vi "chooseParametersFromFiles.vi"(0 "Game in":refnum<class "Game.lvclass">, 1 "MainGameConfigs":T1={"SSL UDP RX"={"Local IP:"="", "Port"=10002, "Server IP:"="224.0.0.1"}, "RefBox UDP RX"={"Local IP:"="", "Port"=10003, "Server IP:"="224.5.23.2"}, "Com UDP"={"UDP GrSim TX"=TRUE, "Address:"="172.31.17.157", "Port:"=20011}, "Command"="Auto", "Goalie"="0", "Side"=enum."Esquerdo", "Team"=enum."Azul"}, 5 "error in (no error)":errorcluster, 7 "ParametersFromFile":T4) -> (14 "Game out":refnum<class "Game.lvclass">, 15 "MainGameConfigs out":T1={"SSL UDP RX"={"Local IP:"="", "Port"=10002, "Server IP:"="224.0.0.1"}, "RefBox UDP RX"={"Local IP:"="", "Port"=10003, "Server IP:"="224.5.23.2"}, "Com UDP"={"UDP GrSim TX"=TRUE, "Address:"="172.31.17.157", "Port:"=20011}, "Command"="Auto", "Goalie"="0", "Side"=enum."Esquerdo", "Team"=enum."Azul"}, 19 "error out":errorcluster)   [LabVIEW 2020, in "Game.lvclass"]
uses:
  Game.lvclass
  ParametersFromFile.ctl
  MainGameConfig.ctl
  Controls/vision_control.ctl
  Controls/ComUDP.ctl
  Utilities_class/Utilities.lvclass
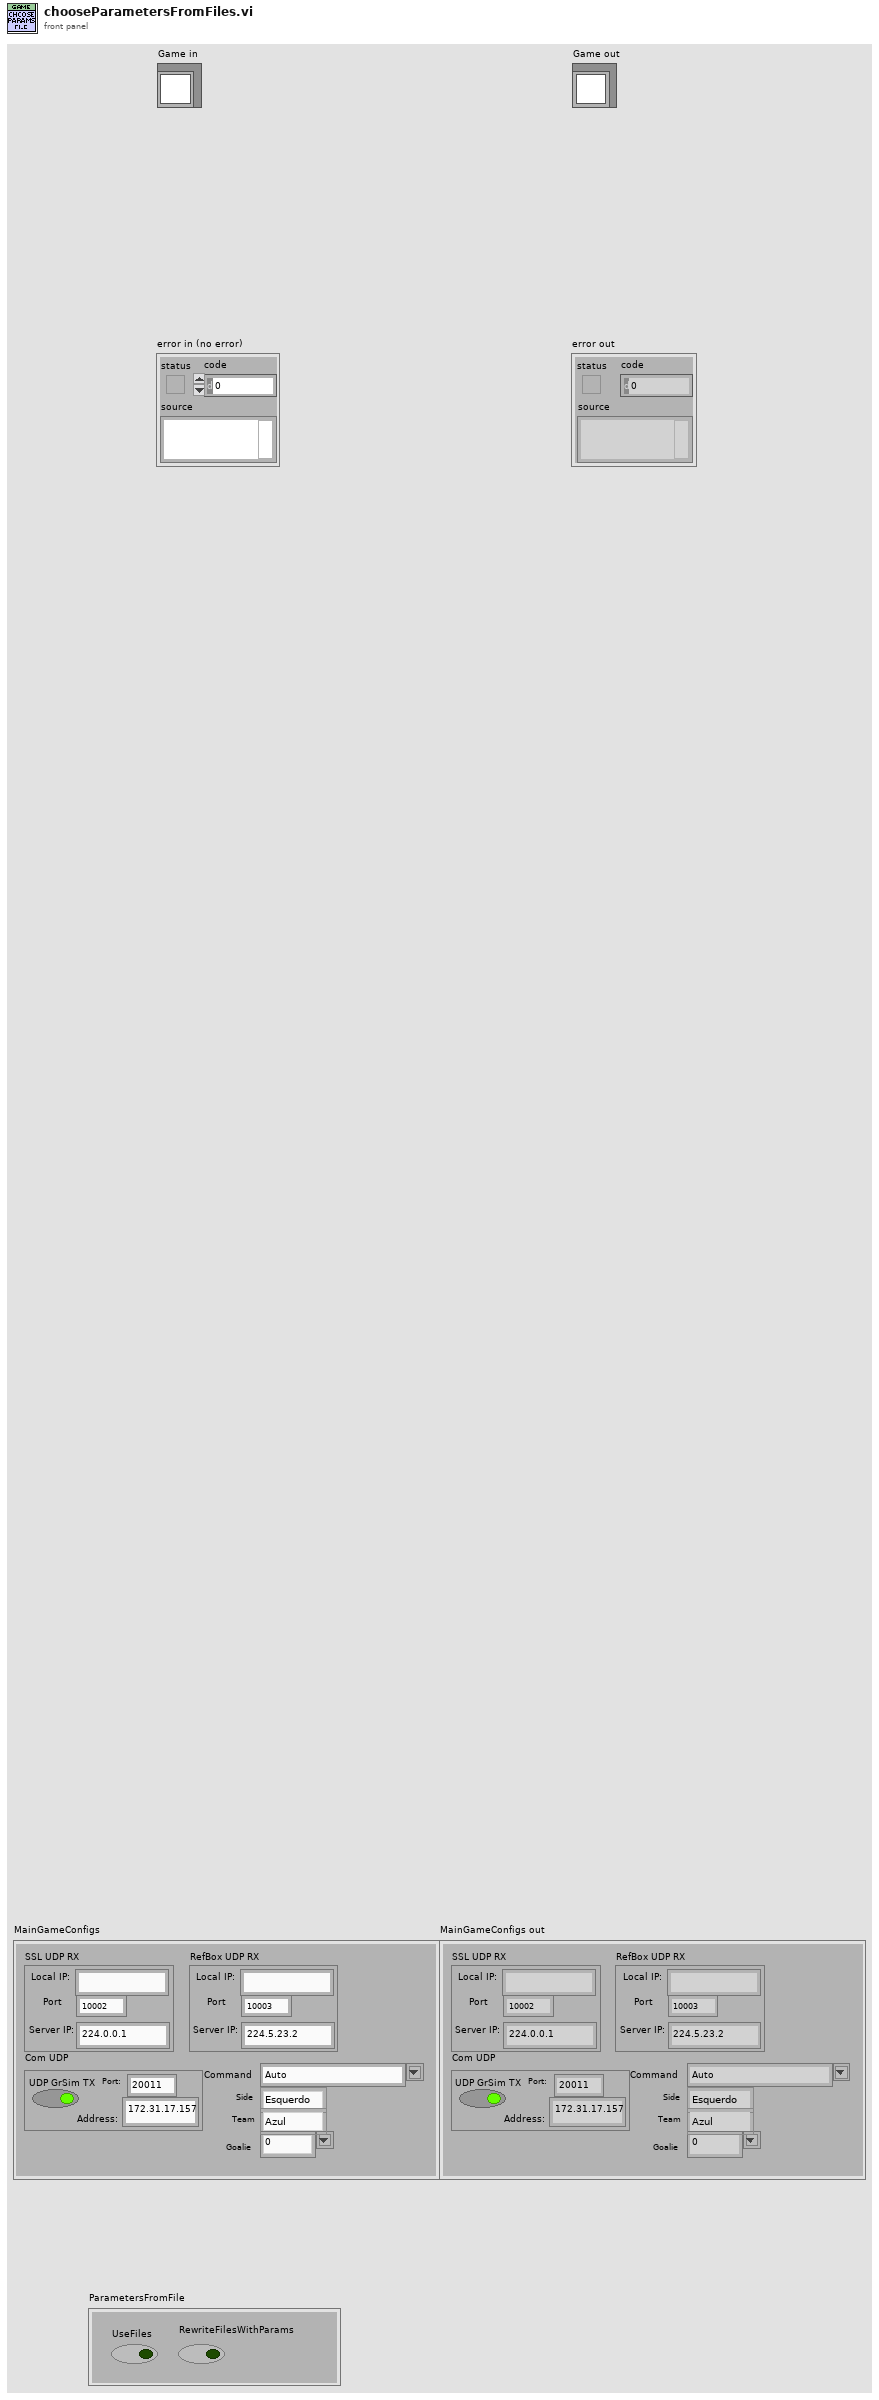
[diagram p1: front panel]
types:
  T1 = typedef "MainGameConfig.ctl" = cluster{"SSL UDP RX":T2, "RefBox UDP RX":T2, "Com UDP":T3, "Command":string, "Goalie":string, "Side":enum16{"Esquerdo", "Direito"}, "Team":enum16{"Azul", "Amarelo"}}
  T2 = typedef "vision_control.ctl" = cluster{"Local IP:":string, "Port":i32, "Server IP:":string}
  T3 = typedef "ComUDP.ctl" = cluster{"UDP GrSim TX":bool, "Address:":string, "Port:":u16}
  T4 = typedef "ParametersFromFile.ctl" = cluster{"UseFiles":bool, "RewriteFilesWithParams":bool}
  T5 = enum16{"open", "replace", "create", "open or create", "replace or create", "replace or create with confirmation"}
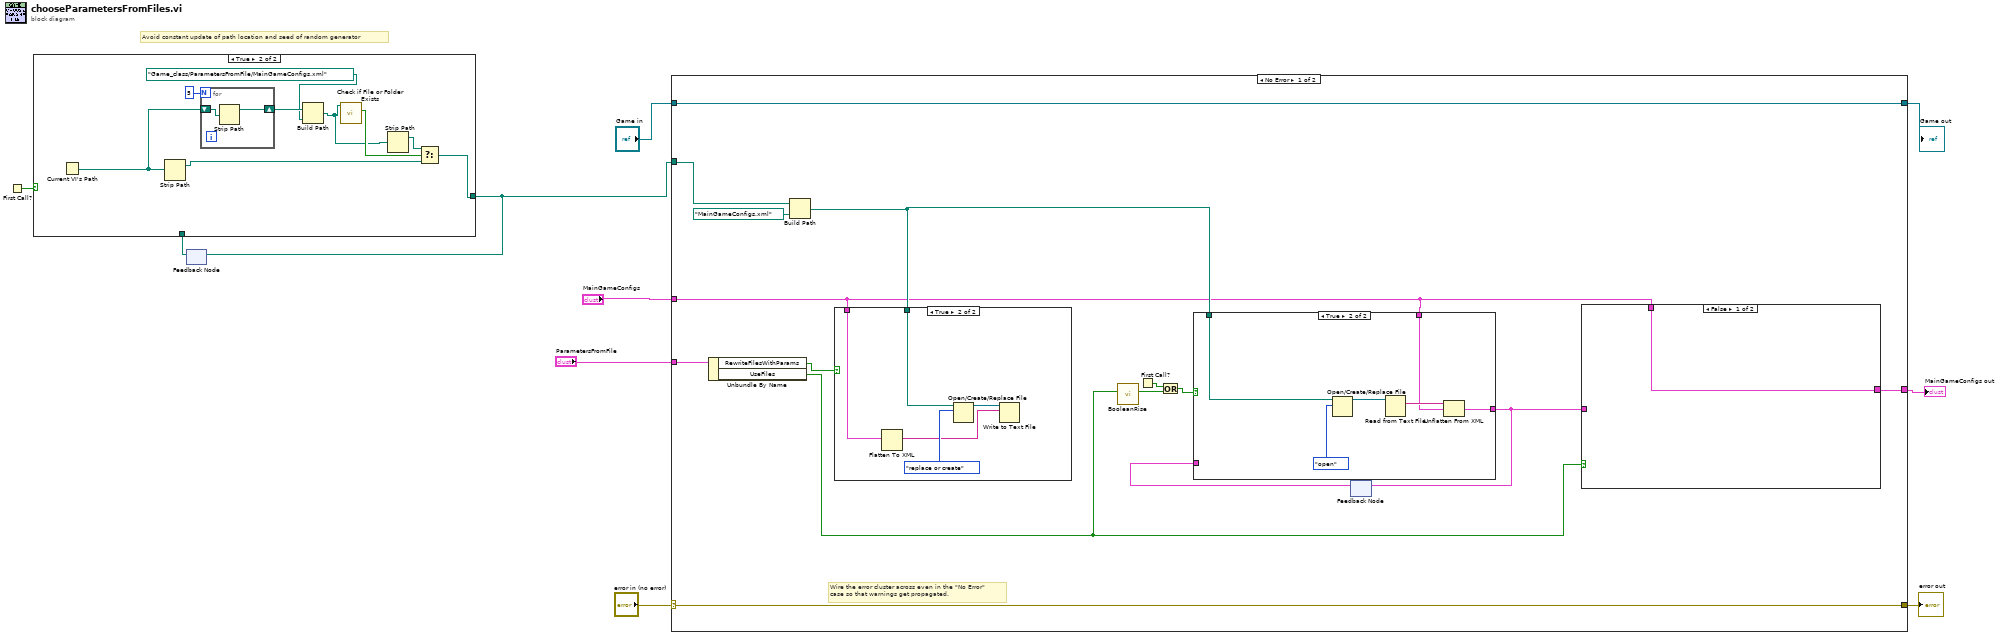
[diagram p0: block diagram]
diagram:
  # "Avoid constant update of path location and seed of random generator"
  n1 = First Call?() -> (First Call?: T/F=w3:bool)
  n2 = feedback #1() -> (w5:path)  [unwired: 1 in]
  n3 = case shown="True" w3 {
    tunnel: [w11 w17] -> w4
    tunnel: w5 -> [w11 _]
    frame False {
    }
    frame True {
      n4 = Current VI's Path() -> (path=w12:path)
      n5 = Strip Path(path=w12) -> (stripped path=w15:path)  [unwired: 1 out]
      n6 = for {
        N: 5 -> [_]
        shift-right: [w21] -> w19
        shift-left: w12 -> [w22]
        n7 = Strip Path(path=w22) -> (stripped path=w21:path)  [unwired: 1 out]
      }
      n8 = Build Path(base path=w19, name or relative path=path "Game_class/ParametersFromFile/MainGameConfigs.xml") -> (appended path=w14:path)
      n9 = call <vilib>:"Check if File or Folder Exists.vi"("path"=w14) -> ("file or folder exists?"=w16:bool)  [unwired: 8 in, 2 out]
      n10 = Strip Path(path=w14) -> (stripped path=w13:path)  [unwired: 1 out]
      n11 = Select(t=w13, s=w16, f=w15) -> (s? t:f=w17:path)
    }
  }
  n12 = feedback-in #1(w4) -> ()
  n13 = case shown="No Error" "error in (no error)" {
    selector: "error in (no error)" -> [w36 w53]
    tunnel: [w36 w53] -> w9
    tunnel: [w37 w52] -> w7
    tunnel: "Game in" -> [w37 w52]
    tunnel: "MainGameConfigs" -> [w29 _]
    tunnel: "ParametersFromFile" -> [w33 _]
    tunnel: w4 -> [w34 _]
    tunnel: [w26 _] -> w1
    frame No Error {
      # "Wire the error cluster across even in the \"No Error\"\ncase so that warnings get propagated."
      n14 = Unbundle By Name(w33) -> ("RewriteFilesWithParams"=w32:bool, "UseFiles"=w31:bool)
      n15 = Build Path(base path=w34, name or relative path=path "MainGameConfigs.xml") -> (appended path=w30:path)
      n16 = case shown="True" w32 {
        tunnel: w29 -> [_ w48]
        tunnel: w30 -> [_ w51]
        frame False {
        }
        frame True {
          n17 = Flatten To XML(6:w48) -> (2:w47:string)
          n18 = Open/Create/Replace File(file path (use dialog)=w51, operation (0:open)=T5."replace or create") -> (refnum out=w49:refnum<file>)  [unwired: 4 in, 2 out]
          n19 = Write to Text File(file (use dialog)=w49, text=w47) -> ()  [unwired: 2 in, 3 out]
        }
      }
      n20 = call "BooleanRise.vi"("Boolean in"=w31) -> ("Boolean"=w24:bool)  [unwired: 8 in, 2 out]
      n21 = First Call?() -> (First Call?: T/F=w25:bool)
      n22 = Or(x=w25, y=w24) -> (x .or. y?=w23:bool)
      n23 = feedback #2() -> (w28:T1)  [unwired: 1 in]
      n24 = case shown="True" w23 {
        tunnel: w30 -> [_ w42]
        tunnel: w29 -> [_ w40]
        tunnel: [w38 w39] -> w27
        tunnel: w28 -> [w38 _]
        frame False {
        }
        frame True {
          n25 = Open/Create/Replace File(file path (use dialog)=w42, operation (0:open)=T5."open") -> (refnum out=w44:refnum<file>)  [unwired: 4 in, 2 out]
          n26 = Read from Text File(file (use dialog)=w44) -> (text=w41:string)  [unwired: 3 in, 3 out]
          n27 = Unflatten From XML(xml string=w41, type=w40) -> (value=w39:T1)  [unwired: 1 in, 1 out]
        }
      }
      n28 = feedback-in #2(w27) -> ()
      n29 = case shown="False" w31 {
        tunnel: w29 -> [w45 _]
        tunnel: [w45 w46] -> w26
        tunnel: w27 -> [_ w46]
        frame False {
        }
        frame True {
        }
      }
    }
    frame Error {
    }
  }
  "error out" <- w9
  "Game out" <- w7
  "MainGameConfigs out" <- w1
